vi "PXIe-7962_FPGA (Host).vi"() -> ()   [LabVIEW 2014]
uses:
  <vilib>/FPGAPlugInAG/PXIe-7962R/niLvFpga_Open_PXIe-7962R.vi
  <vilib>/rvi/interface/common/dynamic/niFpgaDynamicAddResources.vi
  <vilib>/LabVIEW Targets/FPGA/FlexRIO/CustomFPGAMethods/79XXR_Method_IOModuleStatusImpl.vi
  <vilib>/Utility/error.llb/Error Cluster From Error Code.vi
  <vilib>/rvi/errors/niLvFpgaAdjustHostInterfaceError.vi
  <vilib>/rvi/interface/common/niFpgaWaitOnOcc.vi
  <instrlib>/_niInstr/Streaming/v1/Host/Public/Start Finite Stream.vi
  <instrlib>/_niInstr/Streaming/v1/Host/Public/Wait for Stream.vi
  <vilib>/FPGAPlugInAG/Dynamic/niLvFpga_Close_Dynamic.vi
  <vilib>/rvi/interface/nirviOpenFPGA/nirviOpenFPGA.xnode
  FPGA Bitfiles/MochiFPGAControl_FPGATarget_PXIe-7962FPGA_oVYoR0+gQAQ.lvbitx
  <vilib>/rvi/interface/nirviMethod/nirviMethod.xnode
  <vilib>/rvi/interface/nirviReadWriteControl/nirviReadWriteControl.xnode
  <vilib>/rvi/interface/nirviCloseFPGA/nirviCloseFPGA.xnode
  <instrlib>/_niInstr/Streaming/v1/Host/niInstr Streaming v1 Host.lvlib
  <vilib>/rvi/errors/niLvFpgaMergeErrorWithErrorCode.vi
  NiFpgaLv.dll
  <vilib>/rvi/interface/Simulation/niFpgaSimulationCallBeginRW.vi
  <vilib>/FPGAPlugInAG/Dynamic/niLvFpga_ConfigureFifo_Dynamic.vi
  <vilib>/FPGAPlugInAG/Dynamic/niLvFpga_StartFifo_Dynamic.vi
  <vilib>/FPGAPlugInAG/Dynamic/niLvFpga_ReadFifo_Dynamic.vi
panel:
  out "Writes to DMA":i16
  out "Writes to DRAM":i16
  out "Writes to bundeling FIFO":i16
  out "Samples Aquired":i16
  out "Anlog Input 0":dbl[](graph)
  out "Voltage":dbl[][](array[numeric])
  out "Counts":i16[][](array[numeric])
  out "error out":errorcluster
  out "samples transferred":u64
  in  "stop":bool
  out "Raw DMA readout":u64[](array[numeric])
  in  "num samples":u64=1000
  in  "Go":bool
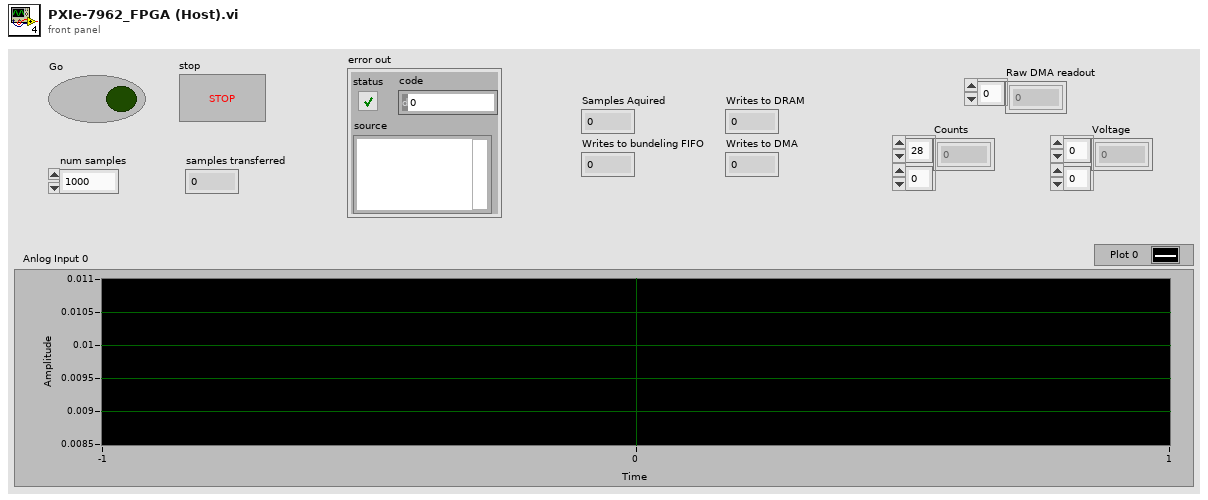
[diagram p1: front panel]
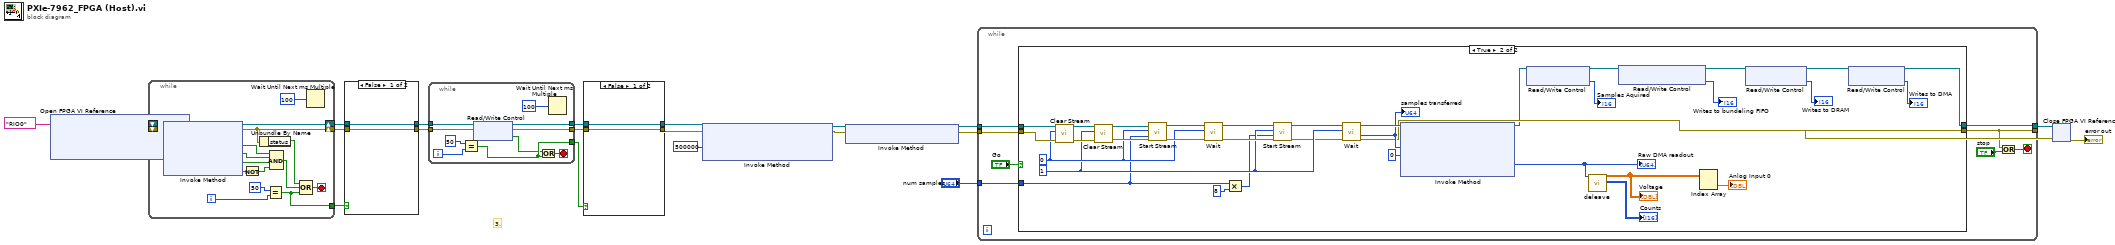
[diagram p0: block diagram]
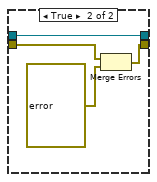
[diagram p2: hidden frame]
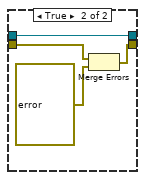
[diagram p3: hidden frame]
diagram:
  # "3."
  n1 = xnode "Open FPGA VI Reference"("resource name"=tag "RIO0") -> ("FPGA VI Reference Out"=w1:refnum<k20>, "error out"=w2:errorcluster)  [unwired: 1 in]
  n2 = while {
    shift-right: [w29] -> w12
    shift-left: w2 -> [w37]
    shift-right: [w36] -> w10
    shift-left: w1 -> [w38]
    tunnel: [w25] -> w11
    i -> [w31]
    stop <- w26 stop-if-true
    n3 = xnode "Invoke Method"("FPGA VI Reference In"=w38, "error in"=w37) -> ("FPGA VI Reference Out"=w36:refnum<k20>, "error out"=w29:errorcluster, "IO Module Present?"=w35:bool, "Power Enabled?"=w34:bool, "IO Enabled?"=w33:bool, "IO Module Mismatch?"=w24:bool)
    n4 = Not(x=w24) -> (.not. x?=w23:bool)
    n5 = Unbundle By Name(w29) -> ("status"=w28:bool)
    n6 = Equal?(x=50, y=w31) -> (x = y?=w25:bool)
    n7 = Compound Arithmetic op=AND(w35, w34, w33, w23) -> (w27:bool)
    n8 = Compound Arithmetic op=OR(w28, w27, w25) -> (w26:bool)
    n9 = Wait Until Next ms Multiple(millisecond multiple=u32 100) -> ()  [unwired: 1 out]
  }
  n10 = case shown="False" w11 {
    tunnel: w12 -> [w39 w43]
    tunnel: [w39 w42] -> w8
    tunnel: w10 -> [w40 w41]
    tunnel: [w40 w41] -> w9
    frame False {
    }
    frame True {
      n11 = Merge Errors(w43, errorcluster {"status"=TRUE, "code"=-1, "source"="The IO Module was not present, powered, or the IO were not enabled.  Verify the NI 5752 is securly connected and try again."} ("error in")) -> (w42:errorcluster)
    }
  }
  n12 = while {
    tunnel: w9 -> [w49]
    tunnel: [w46] -> w7
    tunnel: [w47] -> w6
    tunnel: [w50] -> w5
    tunnel: w8 -> [w48]
    i -> [w53]
    stop <- w51 stop-if-true
    n13 = Equal?(x=50, y=w53) -> (x = y?=w50:bool)
    n14 = xnode "Read/Write Control"("FPGA VI Reference In"=w49, "error in"=w48) -> ("FPGA VI Reference Out"=w46:refnum<k20>, "error out"=w47:errorcluster, "Init Done"=w45:bool)
    n15 = Or(x=w45, y=w50) -> (x .or. y?=w51:bool)
    n16 = Wait Until Next ms Multiple(millisecond multiple=u32 100) -> ()  [unwired: 1 out]
  }
  n17 = case shown="False" w5 {
    tunnel: w6 -> [w55 w59]
    tunnel: [w55 w58] -> w3
    tunnel: w7 -> [w56 w57]
    tunnel: [w56 w57] -> w4
    frame False {
    }
    frame True {
      n18 = Merge Errors(w59, errorcluster {"status"=TRUE, "code"=-1, "source"="The IO Module CLIP was not ready. If you are using any external clocks, make sure they are connected and within the supported specifications."} ("error in")) -> (w58:errorcluster)
    }
  }
  n19 = xnode "Invoke Method"("FPGA VI Reference In"=w4, "error in"=w3, "Requested Depth"=u32 500000) -> ("FPGA VI Reference Out"=w21:refnum<k20>, "error out"=w20:errorcluster)  [unwired: 1 out]
  n20 = xnode "Invoke Method"("FPGA VI Reference In"=w21, "error in"=w20) -> ("FPGA VI Reference Out"=w19:refnum<k20>, "error out"=w18:errorcluster)
  n21 = while {
    tunnel: w19 -> [w67]
    tunnel: w18 -> [w66]
    tunnel: "num samples" -> [w65]
    tunnel: [w64] -> w14
    tunnel: [w62] -> w16
    stop <- w61 stop-if-true
    n22 = case shown="True" "Go" {
      tunnel: w67 -> [w70 w104]
      tunnel: w66 -> [w69 w103]
      tunnel: w65 -> [_ w72]
      tunnel: [w69 w91] -> w62
      tunnel: [w70 w82] -> w64
      frame False {
      }
      frame True {
        w76 = 1 ("stream index")
        w79 = 0 ("stream index")
        n23 = call <instrlib>:"Clear Stream.vi"("error in (no error)"=w103, "stream index"=w79, "refnum in"=w104) -> ("error out"=w101:errorcluster, "refnum out"=w102:refnum<k20>)  [unwired: 7 in]
        n24 = call <instrlib>:"Clear Stream.vi"("error in (no error)"=w101, "stream index"=w76, "refnum in"=w102) -> ("error out"=w99:errorcluster, "refnum out"=w100:refnum<k20>)  [unwired: 7 in]
        n25 = call-poly <instrlib>:"Start Stream.vi"("error in (no error)"=w99, "num samples"=w72, "stream index"=w79, "refnum in"=w100) -> ("error out"=w80:errorcluster, "refnum out"=w81:refnum<k20>)  [unwired: 6 in]
        n26 = call-poly <instrlib>:"Wait.vi"("error in (no error)"=w80, "stream index"=w79, "refnum in"=w81) -> ("error out"=w77:errorcluster, "refnum out"=w78:refnum<k20>)  [unwired: 5 in, 2 out]
        n27 = Multiply(x=w72, y=u64 8) -> (x*y=w73:u64)
        n28 = call-poly <instrlib>:"Start Stream.vi"("error in (no error)"=w77, "num samples"=w73, "stream index"=w76, "refnum in"=w78) -> ("error out"=w74:errorcluster, "refnum out"=w75:refnum<k20>)  [unwired: 6 in]
        n29 = call-poly <instrlib>:"Wait.vi"("error in (no error)"=w74, "stream index"=w76, "refnum in"=w75) -> ("error out"=w91:errorcluster, "samples transferred"=w97:u64, "refnum out"=w98:refnum<k20>)  [unwired: 5 in, 1 out]
        "samples transferred" <- w97
        n30 = xnode "Invoke Method"("FPGA VI Reference In"=w98, "Number of Elements"=w97, "Timeout (ms)"=0) -> ("FPGA VI Reference Out"=w90:refnum<k20>, "Data"=w95:u64[])  [unwired: 1 in, 2 out]
        "Raw DMA readout" <- w95
        n31 = xnode "Read/Write Control"("FPGA VI Reference In"=w90) -> ("FPGA VI Reference Out"=w89:refnum<k20>, "Samples Aquired"=→"Samples Aquired":i16)  [unwired: 1 in, 1 out]
        n32 = call "deleave.vi"("Data"=w95) -> ("Counts"=→"Counts":i16[][], "Voltage"=w93:dbl[][])  [unwired: 9 in]
        "Voltage" <- w93
        n33 = xnode "Read/Write Control"("FPGA VI Reference In"=w89) -> ("FPGA VI Reference Out"=w88:refnum<k20>, "Writes to bundeling FIFO"=→"Writes to bundeling FIFO":i16)  [unwired: 1 in, 1 out]
        n34 = Index Array(array=w93) -> (element=→"Anlog Input 0":dbl[])  [unwired: 2 in]
        n35 = xnode "Read/Write Control"("FPGA VI Reference In"=w88) -> ("FPGA VI Reference Out"=w83:refnum<k20>, "Writes to  DRAM"=→"Writes to DRAM":i16)  [unwired: 1 in, 1 out]
        n36 = xnode "Read/Write Control"("FPGA VI Reference In"=w83) -> ("FPGA VI Reference Out"=w82:refnum<k20>, "Writes to DMA"=→"Writes to DMA":i16)  [unwired: 1 in, 1 out]
      }
    }
    n37 = Or(x=w62, y="stop") -> (x .or. y?=w61:bool)
  }
  n38 = xnode "Close FPGA VI Reference"("FPGA VI Reference In"=w14, "error in"=w16) -> ("error out"=→"error out":errorcluster)
